vi "Groups by Pattern.vi"(8 "error in (no error)":errorcluster, 10 "Group Pattern":string, 11 "ChannelService in":refnum<class "ChannelService.lvclass">) -> (0 "error out":errorcluster, 2 "Node Groups":refnum<class "Group.lvclass">[](array[class]), 3 "ChannelService out":refnum<class "ChannelService.lvclass">)   [LabVIEW 2020, in "Vecto.lvlib" / "ChannelService.lvclass"]
uses:
  ChannelService.lvclass
  Group/Group.lvclass
  GroupsAbstractValue/GroupsAbstractValue.lvclass
  C:/dev/lv20CE/relink/lv-promises/Promises/Value/Value.lvclass
  Lookup Group Data.ctl
  Lookup Type.ctl
  lv-promises/Promises/Promise/Promise.lvclass
  ChannelService.lvclass/ChannelService.ctl
  lv-promises/Promises/Promise/Promise.lvclass/Promise.ctl
  lv-promises/Promises/Future/Future.lvclass/Future.ctl
  GroupsAbstractValue/GroupsAbstractValue.lvclass/GroupsAbstractValue.ctl
  lv-promises/Promises/Future/Future.lvclass
panel:
  in  "Node (All)":string
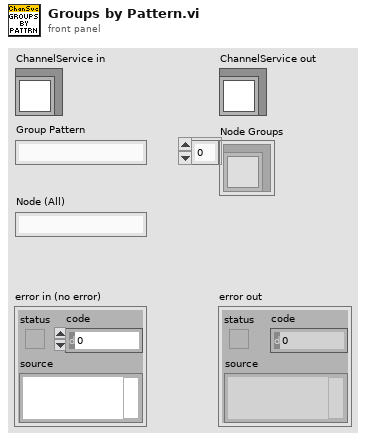
[diagram p1: front panel]
types:
  T1 = typedef "Vecto.lvlib/ChannelService.lvclass/Lookup Type.ctl" = enum16{"Name", "Node", "Pattern"}
  T2 = typedef "Vecto.lvlib/ChannelService.lvclass/Lookup Group Data.ctl" = cluster{"Type":T1, "Group Lookup":string, "Node Lookup":string, "Promise":refnum<class "Promise.lvclass">}
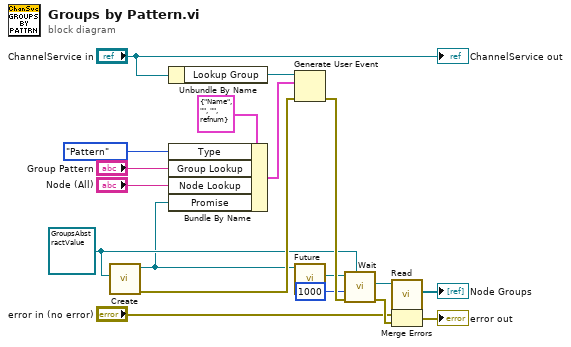
[diagram p0: block diagram]
diagram:
  w12 = refnum<class "GroupsAbstractValue.lvclass"> refnum ("Vecto.lvlib:GroupsValue.lvclass")
  n1 = call "Create.vi"("Result Type"=w12) -> ("error out"=w15:errorcluster, "Promise"=w7:refnum<class "Promise.lvclass">)  [unwired: 9 in]
  n2 = Unbundle By Name("ChannelService in") -> ("Lookup Group"=w14:refnum<user-event>)
  n3 = Bundle By Name(cluster=T2 {"Type"=enum."Name", "Group Lookup"="", "Node Lookup"="", "Promise"=refnum} ("Lookup Group Data"), "Type"=Lookup_Type."Pattern", "Group Lookup"="Group Pattern", "Node Lookup"="Node (All)", "Promise"=w7) -> (w6:T2)
  n4 = Generate User Event(user event=w14, event data cluster=w6, error in=w15) -> (error out=w16:errorcluster)  [unwired: 1 in, 1 out]
  n5 = call "Future.vi"("Promise in"=w7) -> ("Future"=w13:refnum<class "Future.lvclass">)  [unwired: 9 in, 1 out]
  n6 = call "Wait.vi"("Result Type"=w12, "error in (no error)"=w16, "Timeout mS (-1)"=1000, "Future in"=w13) -> ("error out"=w18:errorcluster, "Result"=w10:refnum<class "GroupsAbstractValue.lvclass">)  [unwired: 6 in]
  n7 = call "Read.vi"("GroupsAbstractValue in"=w10) -> ("Groups"=→"Node Groups":refnum<class "Group.lvclass">[])  [unwired: 10 in]
  n8 = Merge Errors("error in (no error)", w18) -> (→"error out":errorcluster)
  "ChannelService out" <- "ChannelService in"
